vi "Initialize COMM VI.vi"(8 "error in (no error)":errorcluster, 11 "Roda_Filtros in":refnum<class "Roda_Filtros.lvclass">) -> (0 "error out":errorcluster, 3 "Roda_Filtros out":refnum<class "Roda_Filtros.lvclass">)   [LabVIEW 2018, in "Roda_Filtros.lvclass"]
uses:
  Roda_Filtros.lvclass
  Roda_Filtros.lvclass/Roda_Filtros.ctl
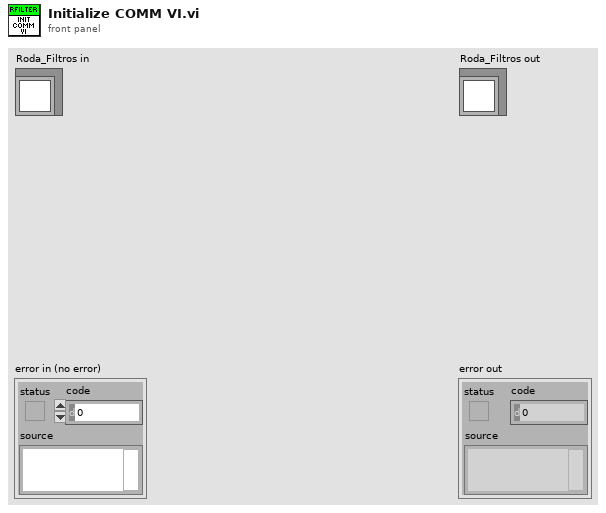
[diagram p1: front panel]
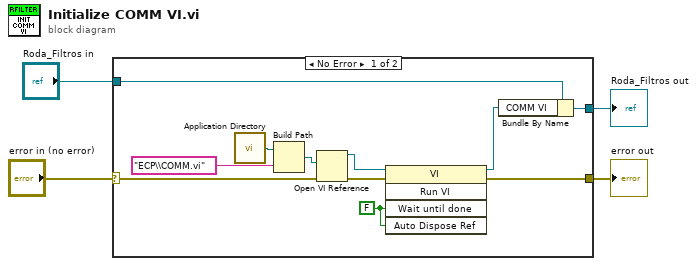
[diagram p0: block diagram]
diagram:
  n1 = case shown="No Error" "error in (no error)" {
    selector: "error in (no error)" -> [w12 w17]
    tunnel: [w11 w17] -> w3
    tunnel: [w9 w16] -> w1
    tunnel: "Roda_Filtros in" -> [w10 w16]
    frame No Error {
      w14 = FALSE ("Wait Until Done")
      n2 = call <vilib>:"Application Directory.vi"() -> ("Application Directory"=w7:path)
      n3 = Build Path(base path=w7, name or relative path="ECP\\COMM.vi") -> (appended path=w5:path)
      n4 = Open VI Reference(vi path=w5, error in (no error)=w12) -> (vi reference=w15:refnum<vi>, error out=w13:errorcluster)  [unwired: 4 in]
      n5 = invoke class="VI" method="Run VI"(reference=w15, error in=w13, "Wait until done"=w14, "Auto Dispose Ref"=w14) -> (reference out=w8:refnum<vi>, error out=w11:errorcluster)  [unwired: 1 in, 3 out]
      n6 = Bundle By Name(cluster=w10, "COMM VI"=w8) -> (w9:refnum<class "Roda_Filtros.lvclass">)
    }
    frame Error {
    }
  }
  "error out" <- w3
  "Roda_Filtros out" <- w1
